vi "pionowy.vi"(6 "error in":errorcluster, 7 "Wybór komory":T1, 8 "Akcja":T8=enum."Reset ramienia", 9 "LINX Resource in":T2) -> (0 "error out":errorcluster, 1 "KONIEC":bool, 2 "Aktualny stan":T9, 3 "LINX Resource out":T2)   [LabVIEW 2014]
uses:
  pionowyVIs/RuchPionowy.ctl
  wczytajDaneDoRuchuVIs/Akcje_wczytywania_danych_do_ruchu.ctl
  <vilib>/MakerHub/LINX/Private/Type Defs/LINX Ref.ctl
  <vilib>/MakerHub/LINX/Private/Type Defs/Platform.ctl
  <vilib>/MakerHub/LINX/Private/Type Defs/Interface.ctl
  <vilib>/MakerHub/LINX/Private/Device/Type Defs/LINX Device Config.ctl
  <vilib>/MakerHub/LINX/Private/Device/Type Defs/TCP Config.ctl
  <vilib>/MakerHub/LINX/Private/Device/Type Defs/Channels.ctl
  parametryKomorVIs/WyborKomory.ctl
  Faza_ruchu.ctl
  wczytaj_zapisz.ctl
  pionowyVIs/akcelerometrVIs/czytajI2CVIs/usrednijVIs/AkcjaUsredniania.ctl
  pionowyVIs/ParametryRuchyPionowego.ctl
  <vilib>/MakerHub/LINX/LMH-LINX.lvlib
  <vilib>/MakerHub/LINX/Private/Device/Device.lvlib
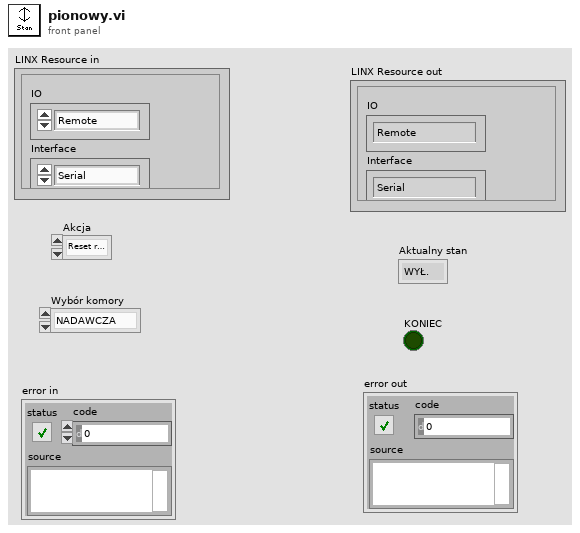
[diagram p1: front panel]
types:
  T1 = typedef "WyborKomory.ctl" = enum16{"NADAWCZA", "ODBIORCZA"}
  T2 = typedef "LMH-LINX.lvlib/LINX Ref.ctl" = cluster{"IO":T3, "Interface":T4, "LINX Device Config":T5}
  T3 = typedef "LMH-LINX.lvlib/Platform.ctl" = enum16{"Remote", "Local"}
  T4 = typedef "LMH-LINX.lvlib/Interface.ctl" = enum16{"Serial", "TCP"}
  T5 = typedef "LMH-LINX.lvlib/Device.lvlib/LINX Device Config.ctl" = cluster{"Interface":T4, "COM Port":refnum<visa-resource-name>, "TCP Configuration":T6, "Device Family":u8, "Device ID":u8, "Device Name":string, "TCP Ref":refnum<k5>, "Channels":T7}
  T6 = typedef "LMH-LINX.lvlib/Device.lvlib/TCP Config.ctl" = cluster{"IP Address":string, "Port":u16}
  T7 = typedef "LMH-LINX.lvlib/Channels.ctl" = cluster{"DI":u8[], "DO":u8[], "AI":u8[], "AO":u8[], "PWM":u8[], "QE":u8[], "UART":u8[], "I2C 2":u8[], "SPI":u8[], "CAN":u8[], "Servo":u8[], "AI Ref (V)":dbl, "AI Resolution (Bits)":u8, "AO Ref (V)":dbl, "AO Resolution (Bits)":u8}
  T8 = typedef "Akcje_wczytywania_danych_do_ruchu.ctl" = enum16{"Init", "Reset ramienia", "Przygotuj listę", "Sprawdź", "Koniec"}
  T9 = typedef "RuchPionowy.ctl" = enum16{"WYŁ.", "GÓRA", "Dӣ", "PRACA RĘCZNA"}
  T10 = typedef "wczytaj_zapisz.ctl" = enum16{"Zapisz", "Wczytaj"}
  T11 = typedef "Faza_ruchu.ctl" = enum16{"Ruch", "Poczekaj", "Pomiar"}
  T12 = typedef "AkcjaUsredniania.ctl" = enum16{"Init", "DodajWartość", "WypełnijKolejkę", "Czyść"}
  T13 = typedef "ParametryRuchyPionowego.ctl" = cluster{"Faza ruchu":T11, "Lista punktów w pionie":i32[], "Adres I2C":u8}
  T14 = typedef "Gotowosc.ctl" = cluster{"Poziomy":bool, "Pionowy":bool}
  T15 = typedef "Przyciski_zbior.ctl" = cluster{"LEWO":bool, "PRAWO":bool, "GÓRA":bool, "Dӣ":bool, "Stop":bool, "Start":bool, "Praca ręczna":bool, "Komora":bool}
  T16 = typedef "PinoutLista.ctl" = cluster{"LEWO":u8, "PRAWO":u8, "GÓRA":u8, "Dӣ":u8, "CZUJNIK":u8, "I2C ADRES":u8}
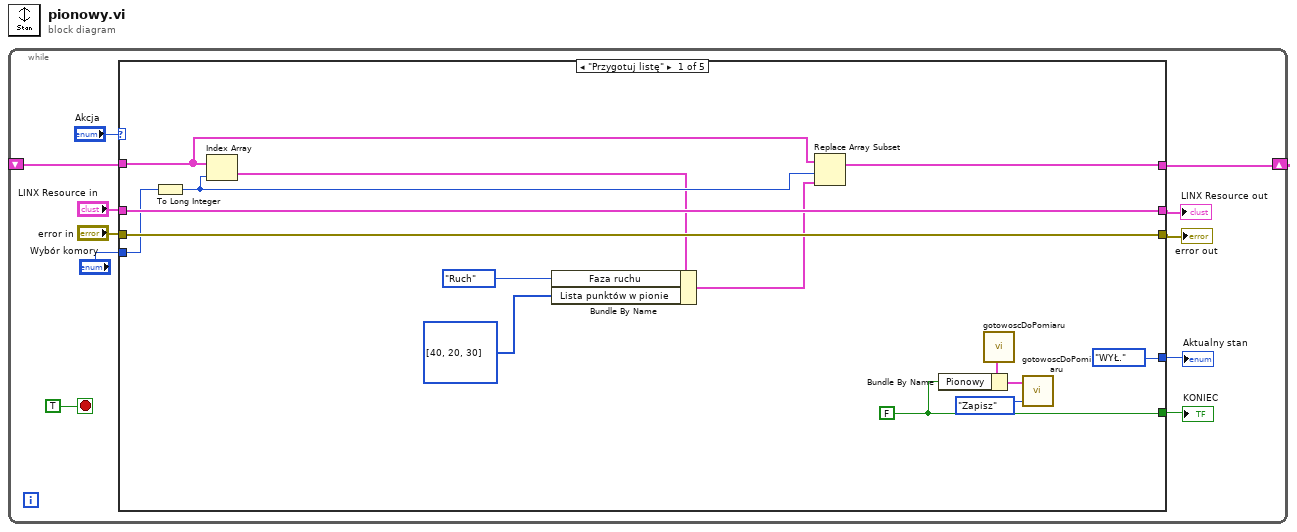
[diagram p0: block diagram]
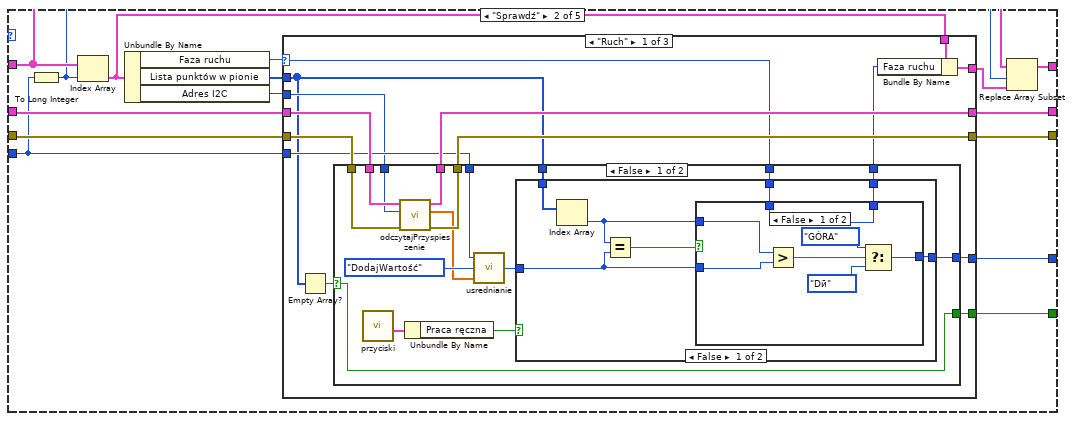
[diagram p2: hidden frame]
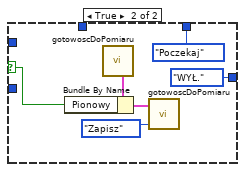
[diagram p3: hidden frame]
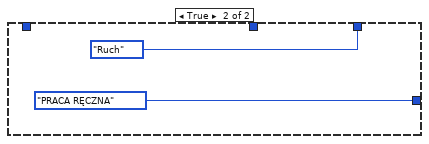
[diagram p4: hidden frame]
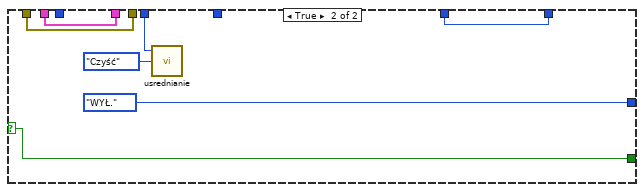
[diagram p5: hidden frame]
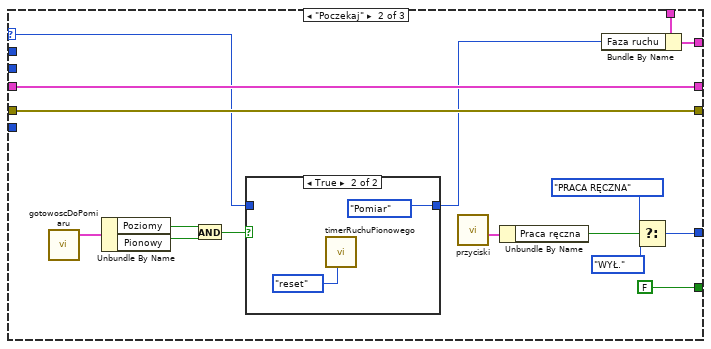
[diagram p6: hidden frame]
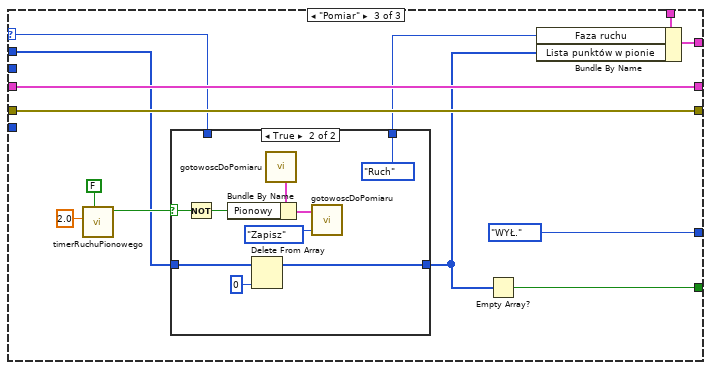
[diagram p8: hidden frame]
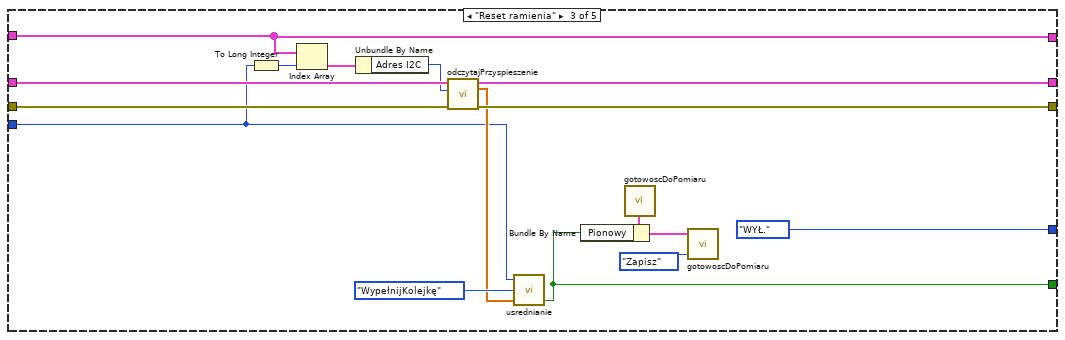
[diagram p10: hidden frame]
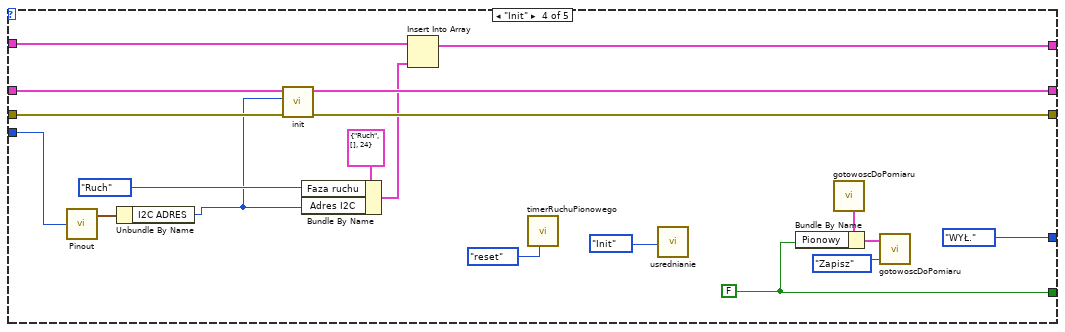
[diagram p11: hidden frame]
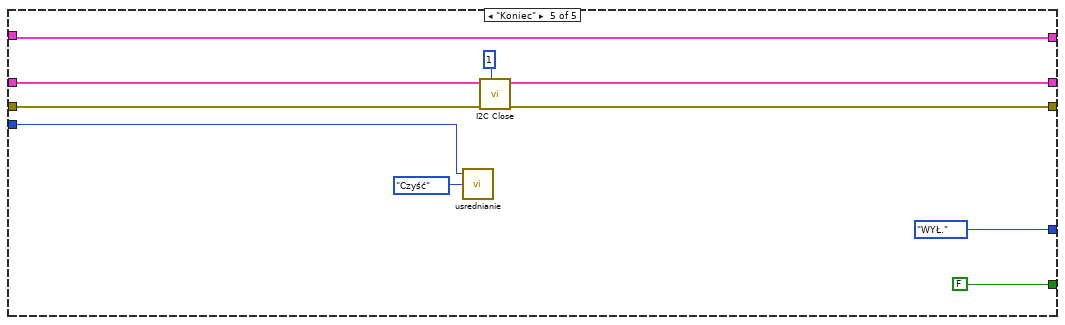
[diagram p12: hidden frame]
diagram:
  n1 = while {
    shift-right: [w10] -> _
    shift-left: _ -> [w7]
    stop <- TRUE stop-if-true
    n2 = case shown="\"Przygotuj listę\"" "Akcja" {
      tunnel: "error in" -> [w25 w40 w152 w172 w187]
      tunnel: [w25 w38 w150 w170 w184] -> w3
      tunnel: [w26 w39 w151 w171 w185] -> w4
      tunnel: "LINX Resource in" -> [w26 w41 w153 w173 w188]
      tunnel: [w20 w36 w155 w169 FALSE ("empty?")] -> w1
      tunnel: [RuchPionowy."WYŁ." ("Aktualny stan") w37 RuchPionowy."WYŁ." ("Aktualny stan") RuchPionowy."WYŁ." ("Aktualny stan") RuchPionowy."WYŁ." ("Aktualny stan")] -> w2
      tunnel: "Wybór komory" -> [w15 w35 w147 w162 w180]
      tunnel: [w17 w30 w144 w164 w179] -> w10
      tunnel: w7 -> [w12 w31 w144 w165 w179]
      frame "Przygotuj listę" {
        w20 = FALSE ("Poziomy")
        n3 = To Long Integer(number=w15) -> (32bit integer=w14:i32)
        n4 = Index Array(array=w12, index=w14) -> (element=w13:T13)
        n5 = Bundle By Name(cluster=w13, "Faza ruchu"=Faza_ruchu."Ruch", "Lista punktów w pionie"=i32[] [40, 20, 30]) -> (w16:T13)
        n6 = Replace Array Subset(array=w12, new element=w16, index=w14) -> (w17:T13[])
        n7 = call "gotowoscDoPomiaru.vi"() -> ("Gotowość wyjście"=w22:T14)  [unwired: 5 in]
        n8 = Bundle By Name(cluster=w22, "Pionowy"=w20) -> (w23:T14)
        n9 = call "gotowoscDoPomiaru.vi"("Wczytaj_zapisz"=wczytaj_zapisz."Zapisz", "Gotowość"=w23) -> ()  [unwired: 3 in, 1 out]
      }
      frame "Sprawdź" {
        n10 = To Long Integer(number=w35) -> (32bit integer=w28:i32)
        n11 = Index Array(array=w31, index=w28) -> (element=w27:T13)
        n12 = Unbundle By Name(w27) -> ("Faza ruchu"=w34:T11, "Lista punktów w pionie"=w33:i32[], "Adres I2C"=w32:u8)
        n13 = case shown="\"Ruch\"" w34 {
          selector: w34 -> [w50 w110 w126]
          tunnel: w41 -> [w54 w112 w132]
          tunnel: w40 -> [w55 w111 w131]
          tunnel: [w52 w111 w131] -> w38
          tunnel: [w53 w112 w132] -> w39
          tunnel: [w51 w106 RuchPionowy."WYŁ." ("Stan pionowy")] -> w37
          tunnel: [w48 FALSE ("empty?") w125] -> w36
          tunnel: w35 -> [w47 _ _]
          tunnel: w33 -> [w43 _ w124]
          tunnel: w32 -> [w46 _ _]
          tunnel: [w44 w102 w121] -> w29
          tunnel: w27 -> [w42 w101 w120]
          frame "Ruch" {
            n14 = Empty Array?(array=w43) -> (empty?=w49:bool)
            n15 = case shown="False" w49 {
              selector: w49 -> [w56 w95]
              tunnel: w55 -> [w64 w99]
              tunnel: w54 -> [w61 w100]
              tunnel: [w62 w100] -> w53
              tunnel: [w63 w99] -> w52
              tunnel: [w67 RuchPionowy."WYŁ." ("Stan pionowy")] -> w51
              tunnel: w50 -> [w66 w98]
              tunnel: [w65 w98] -> w45
              tunnel: [w56 w95] -> w48
              tunnel: w46 -> [w60 _]
              tunnel: w47 -> [w59 w94]
              tunnel: w43 -> [w58 _]
              frame False {
                n16 = call "przyciski.vi"() -> ("Wyjście"=w69:T15)  [unwired: 5 in]
                n17 = call "odczytajPrzyspieszenie.vi"("Error In"=w64, "I2C Adres"=w60, "LINX Resource"=w61) -> ("Error Out"=w63:errorcluster, "Kąty nachylenia (st.)"=w57:dbl[], "LINX Resource 2"=w62:T2)  [unwired: 6 in]
                n18 = Unbundle By Name(w69) -> ("Praca ręczna"=w68:bool)
                n19 = call "usrednianie.vi"("Wartości"=w57, "AkcjaUsredniania"=AkcjaUsredniania."DodajWartość", "Wybór Komory"=w59) -> ("Przysp. uśrednione"=w70:i32)  [unwired: 1 in, 1 out]
                n20 = case shown="False" w68 {
                  tunnel: w70 -> [w74 _]
                  tunnel: [w76 RuchPionowy."PRACA RĘCZNA" ("Stan pionowy")] -> w67
                  tunnel: w66 -> [w77 _]
                  tunnel: [w78 Faza_ruchu."Ruch" ("Faza ruchu")] -> w65
                  tunnel: w58 -> [w73 _]
                  frame False {
                    n21 = Index Array(array=w73) -> (element=w72:i32)  [unwired: 1 in]
                    n22 = Equal?(x=w72, y=w74) -> (x = y?=w75:bool)
                    n23 = case shown="False" w75 {
                      selector: w75 -> [_ w86]
                      tunnel: [w85 Faza_ruchu."Poczekaj" ("t")] -> w78
                      tunnel: w77 -> [w85 _]
                      tunnel: [w80 RuchPionowy."WYŁ." ("Stan pionowy")] -> w76
                      tunnel: w74 -> [w84 _]
                      tunnel: w72 -> [w79 _]
                      frame False {
                        n24 = Greater?(x=w79, y=w84) -> (0:w83:bool)
                        n25 = Select(t=RuchPionowy."GÓRA" ("Stan pionowy"), s=w83, f=RuchPionowy."Dӣ") -> (s? t:f=w80:T9)
                      }
                      frame True {
                        n26 = call "gotowoscDoPomiaru.vi"() -> ("Gotowość wyjście"=w88:T14)  [unwired: 5 in]
                        n27 = Bundle By Name(cluster=w88, "Pionowy"=w86) -> (w89:T14)
                        n28 = call "gotowoscDoPomiaru.vi"("Wczytaj_zapisz"=wczytaj_zapisz."Zapisz", "Gotowość"=w89) -> ()  [unwired: 3 in, 1 out]
                      }
                    }
                  }
                  frame True {
                  }
                }
              }
              frame True {
                n29 = call "usrednianie.vi"("AkcjaUsredniania"=AkcjaUsredniania."Czyść", "Wybór Komory"=w94) -> ()  [unwired: 2 in, 2 out]
              }
            }
            n30 = Bundle By Name(cluster=w42, "Faza ruchu"=w45) -> (w44:T13)
          }
          frame "Poczekaj" {
            n31 = call "gotowoscDoPomiaru.vi"() -> ("Gotowość wyjście"=w114:T14)  [unwired: 5 in]
            n32 = Unbundle By Name(w114) -> ("Poziomy"=w116:bool, "Pionowy"=w115:bool)
            n33 = And(x=w116, y=w115) -> (x .and. y?=w113:bool)
            n34 = case shown="True" w113 {
              tunnel: w110 -> [w117 _]
              tunnel: [w117 Faza_ruchu."Pomiar" ("t")] -> w103
              frame False {
              }
              frame True {
                n35 = call "timerRuchuPionowego.vi"("Czynność"=enum16{"reset", "działaj"}."reset") -> ()  [unwired: 10 in, 1 out]
              }
            }
            n36 = call "przyciski.vi"() -> ("Wyjście"=w109:T15)  [unwired: 5 in]
            n37 = Unbundle By Name(w109) -> ("Praca ręczna"=w107:bool)
            n38 = Bundle By Name(cluster=w101, "Faza ruchu"=w103) -> (w102:T13)
            n39 = Select(t=RuchPionowy."PRACA RĘCZNA", s=w107, f=RuchPionowy."WYŁ." ("Stan pionowy")) -> (s? t:f=w106:T9)
          }
          frame "Pomiar" {
            n40 = call "timerRuchuPionowego.vi"("pauza"=FALSE, "Czas"=2.0) -> ("czy czas upłynął"=w130:bool)  [unwired: 9 in]
            n41 = case shown="True" w130 {
              selector: w130 -> [_ w136]
              tunnel: [w133 w143] -> w122
              tunnel: w126 -> [w134 _]
              tunnel: [w134 Faza_ruchu."Ruch" ("Faza ruchu")] -> w123
              tunnel: w124 -> [w133 w137]
              frame False {
              }
              frame True {
                n42 = Not(x=w136) -> (.not. x?=w135:bool)
                n43 = Delete From Array(array=w137, index=0) -> (array with subset deleted=w143:i32[])  [unwired: 1 in, 1 out]
                n44 = call "gotowoscDoPomiaru.vi"() -> ("Gotowość wyjście"=w139:T14)  [unwired: 5 in]
                n45 = Bundle By Name(cluster=w139, "Pionowy"=w135) -> (w140:T14)
                n46 = call "gotowoscDoPomiaru.vi"("Wczytaj_zapisz"=wczytaj_zapisz."Zapisz", "Gotowość"=w140) -> ()  [unwired: 3 in, 1 out]
              }
            }
            n47 = Empty Array?(array=w122) -> (empty?=w125:bool)
            n48 = Bundle By Name(cluster=w120, "Faza ruchu"=w123, "Lista punktów w pionie"=w122) -> (w121:T13)
          }
        }
        n49 = Replace Array Subset(array=w31, new element=w29, index=w28) -> (w30:T13[])
      }
      frame "Reset ramienia" {
        n50 = To Long Integer(number=w147) -> (32bit integer=w146:i32)
        n51 = Index Array(array=w144, index=w146) -> (element=w145:T13)
        n52 = Unbundle By Name(w145) -> ("Adres I2C"=w148:u8)
        n53 = call "odczytajPrzyspieszenie.vi"("Error In"=w152, "I2C Adres"=w148, "LINX Resource"=w153) -> ("Error Out"=w150:errorcluster, "Kąty nachylenia (st.)"=w149:dbl[], "LINX Resource 2"=w151:T2)  [unwired: 6 in]
        n54 = call "usrednianie.vi"("Wartości"=w149, "AkcjaUsredniania"=AkcjaUsredniania."WypełnijKolejkę", "Wybór Komory"=w147) -> ("Czy kolejka pełna?"=w155:bool)  [unwired: 1 in, 1 out]
        n55 = call "gotowoscDoPomiaru.vi"() -> ("Gotowość wyjście"=w158:T14)  [unwired: 5 in]
        n56 = Bundle By Name(cluster=w158, "Pionowy"=w155) -> (w157:T14)
        n57 = call "gotowoscDoPomiaru.vi"("Wczytaj_zapisz"=wczytaj_zapisz."Zapisz", "Gotowość"=w157) -> ()  [unwired: 3 in, 1 out]
      }
      frame "Init" {
        w169 = FALSE ("Poziomy")
        n58 = call "Pinout.vi"("Wybór komory"=w162) -> ("Wyjście"=w161:T16)  [unwired: 4 in]
        n59 = Unbundle By Name(w161) -> ("I2C ADRES"=w160:u8)
        n60 = call "init.vi"("Error In"=w172, "I2C Adres"=w160, "LINX Ref"=w173) -> ("Error Out"=w170:errorcluster, "LINX Resource"=w171:T2)  [unwired: 7 in]
        n61 = Bundle By Name(cluster=T13 {"Faza ruchu"=enum."Ruch", "Lista punktów w pionie"=[], "Adres I2C"=24} ("Parametry ruchy pionowego"), "Faza ruchu"=Faza_ruchu."Ruch", "Adres I2C"=w160) -> (w163:T13)
        n62 = Insert Into Array(array=w165, new element=w163) -> (w164:T13[])  [unwired: 1 in]
        n63 = call "timerRuchuPionowego.vi"("Czynność"=enum16{"reset", "działaj"}."reset") -> ()  [unwired: 10 in, 1 out]
        n64 = call "usrednianie.vi"("AkcjaUsredniania"=AkcjaUsredniania."Init") -> ()  [unwired: 3 in, 2 out]
        n65 = call "gotowoscDoPomiaru.vi"() -> ("Gotowość wyjście"=w175:T14)  [unwired: 5 in]
        n66 = Bundle By Name(cluster=w175, "Pionowy"=w169) -> (w176:T14)
        n67 = call "gotowoscDoPomiaru.vi"("Wczytaj_zapisz"=wczytaj_zapisz."Zapisz", "Gotowość"=w176) -> ()  [unwired: 3 in, 1 out]
      }
      frame "Koniec" {
        n68 = call "usrednianie.vi"("AkcjaUsredniania"=AkcjaUsredniania."Czyść", "Wybór Komory"=w180) -> ()  [unwired: 2 in, 2 out]
        n69 = call <vilib>:"I2C Close.vi"("I2C Channel (0)"=u8 1, "Error In"=w187, "LINX Resource"=w188) -> ("Error Out"=w184:errorcluster, "LINX Resource"=w185:T2)  [unwired: 7 in]
      }
    }
    "error out" <- w3
    "LINX Resource out" <- w4
    "KONIEC" <- w1
    "Aktualny stan" <- w2
  }
